vi "Data to Knobs Present.vi"(7 "String":string="00 00 00 00 00 00 0F FF 00 00 0F FF 00 00 00 00 0F FF 00 00 0F FF 00 00 01 A1 0C B0 00 00 00 00 08 12", 11 "Error In":errorcluster) -> (8 "Knobs Present":bool[](array[boolean]), 15 "Error Out":errorcluster)   [LabVIEW 2016]
panel:
  # "00 00 00 00 00 00 02 63 00 00 07 17 00 00 00 00 04 A3 00 00 09 73 00 00 01 A1 0C E1 00 00 00 00 08 14"
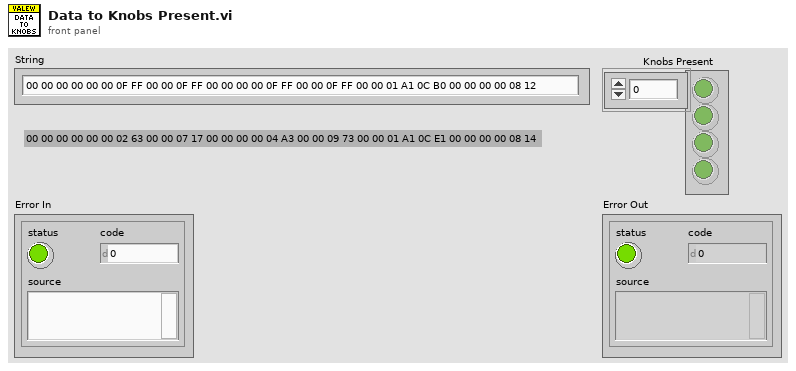
[diagram p1: front panel]
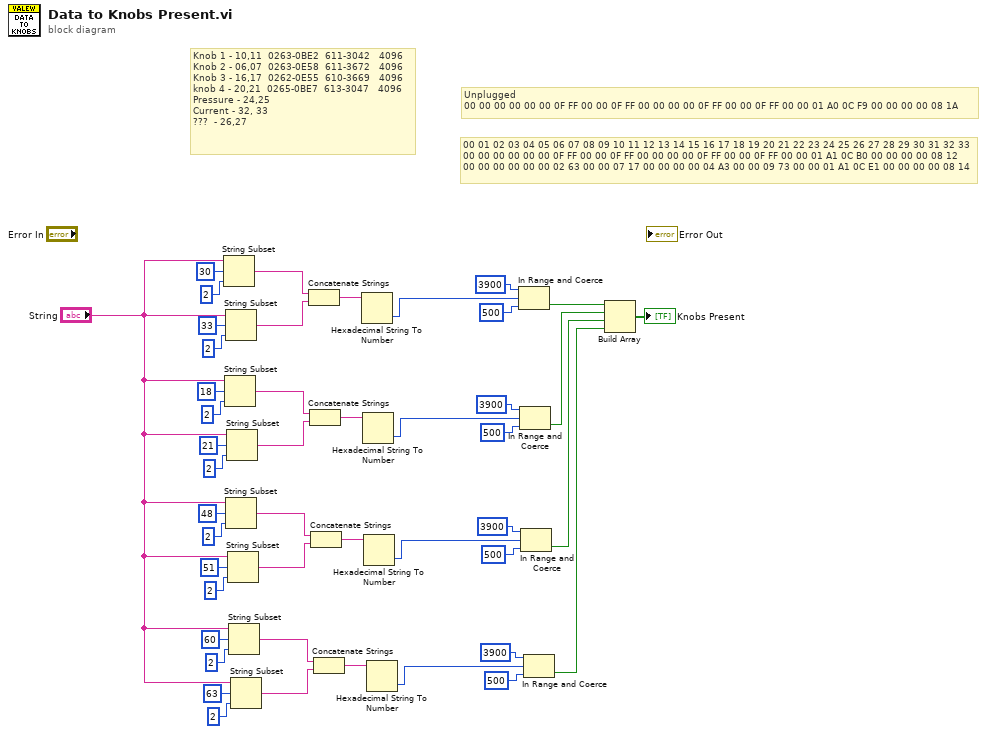
[diagram p0: block diagram]
diagram:
  # "00 01 02 03 04 05 06 07 08 09 10 11 12 13 14 15 16 17 18 19 20 21 22 23 24 25 26 27 28 29 30 31 32 33\n00 00 00 00 00 00 0F FF 00 00 0F FF 00 00 00 00 0F FF 00 00 0F FF 00 00 01 A1 0C B0 00 00 00 00 08 12\n00 00 00 00 00 00 02 63 00 00 07 17 00 00 00 00 04 A3 00 00 09 73 00 00 01 A1 0C E1 00 00 00 00 08 14"
  # "Unplugged\n00 00 00 00 00 00 0F FF 00 00 0F FF 00 00 00 00 0F FF 00 00 0F FF 00 00 01 A0 0C F9 00 00 00 00 08 1A"
  # "Knob 1 - 10,11  0263-0BE2  611-3042   4096\nKnob 2 - 06,07  0263-0E58  611-3672   4096\nKnob 3 - 16,17  0262-0E55  610-3669   4096\nknob 4 - 20,21  0265-0BE7  613-3047   4096\nPressure - 24,25\nCurrent - 32, 33\n???  - 26,27"
  n1 = String Subset(string="String", offset (0)=30, length (rest)=2 ("length (rest)")) -> (substring=w42:string)
  n2 = String Subset(string="String", offset (0)=18, length (rest)=2 ("length (rest)")) -> (substring=w30:string)
  n3 = String Subset(string="String", offset (0)=33, length (rest)=2 ("length (rest)")) -> (substring=w41:string)
  n4 = String Subset(string="String", offset (0)=48, length (rest)=2 ("length (rest)")) -> (substring=w21:string)
  n5 = String Subset(string="String", offset (0)=21, length (rest)=2 ("length (rest)")) -> (substring=w31:string)
  n6 = String Subset(string="String", offset (0)=51, length (rest)=2 ("length (rest)")) -> (substring=w20:string)
  n7 = String Subset(string="String", offset (0)=60, length (rest)=2 ("length (rest)")) -> (substring=w10:string)
  n8 = String Subset(string="String", offset (0)=63, length (rest)=2 ("length (rest)")) -> (substring=w11:string)
  n9 = Concatenate Strings(w42, w41) -> (w40:string)
  n10 = Concatenate Strings(w30, w31) -> (w32:string)
  n11 = Concatenate Strings(w21, w20) -> (w19:string)
  n12 = Concatenate Strings(w10, w11) -> (w12:string)
  n13 = Hexadecimal String To Number(string=w40) -> (number=w39:u32)  [unwired: 2 in, 1 out]
  n14 = Hexadecimal String To Number(string=w32) -> (number=w33:u32)  [unwired: 2 in, 1 out]
  n15 = Hexadecimal String To Number(string=w19) -> (number=w18:u32)  [unwired: 2 in, 1 out]
  n16 = Hexadecimal String To Number(string=w12) -> (number=w13:u32)  [unwired: 2 in, 1 out]
  n17 = In Range and Coerce(upper limit=u32 3900, x=w39, lower limit=u32 500) -> (In Range?=w36:bool)  [unwired: 1 out]
  n18 = In Range and Coerce(upper limit=u32 3900, x=w33, lower limit=u32 500) -> (In Range?=w5:bool)  [unwired: 1 out]
  n19 = In Range and Coerce(upper limit=u32 3900, x=w18, lower limit=u32 500) -> (In Range?=w4:bool)  [unwired: 1 out]
  n20 = In Range and Coerce(upper limit=u32 3900, x=w13, lower limit=u32 500) -> (In Range?=w3:bool)  [unwired: 1 out]
  n21 = Build Array(w36, w5, w4, w3) -> (→"Knobs Present":bool[])
